vi "comunicacion_arduino_ejemplo.vi"() -> ()   [LabVIEW 2014]
panel:
  out "Waveform Chart":dbl(graph)
  in  "Slide":u8(slide) scale=0.0..255.0
  in  "error in (no error)":errorcluster
  in  "baud rate (9600)":u32=9600
  in  "VISA resource name":refnum<visa-resource-name>
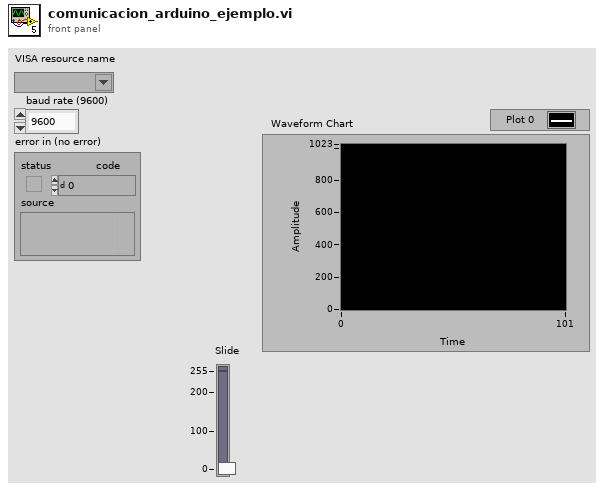
[diagram p1: front panel]
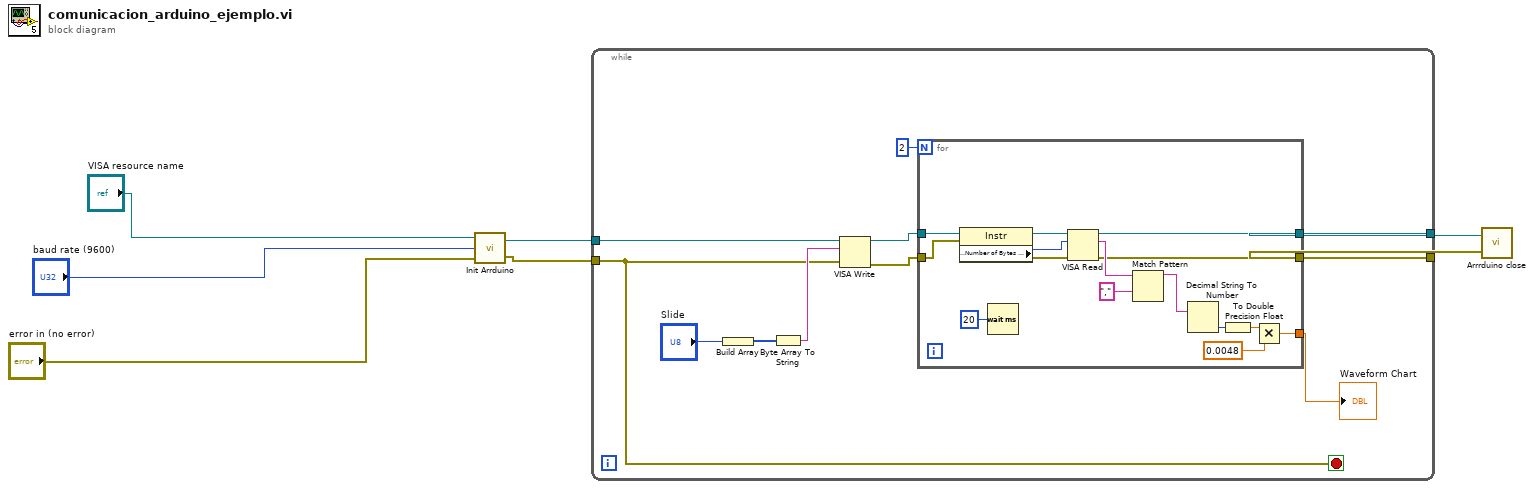
[diagram p0: block diagram]
diagram:
  n1 = call "Init Arrduino.vi"("error in (no error)"="error in (no error)", "baud rate (9600)"="baud rate (9600)", "VISA Refnum in"="VISA resource name") -> ("error out"=w3:errorcluster, "VISA Refnum out"=w4:refnum<visa-resource-name>)
  n2 = while {
    tunnel: w4 -> [w18]
    tunnel: w3 -> [w10]
    tunnel: [w11] -> w2
    tunnel: [w12] -> w1
    stop <- w10 stop-if-true
    n3 = Build Array("Slide") -> (w16:u8[])
    n4 = Byte Array To String(unsigned byte array=w16) -> (string=w15:string)
    n5 = VISA Write(VISA resource name=w18, write buffer=w15, error in (no error)=w10) -> (VISA resource name out=w13:refnum<visa-resource-name>, error out=w14:errorcluster)  [unwired: 1 out]
    n6 = for {
      N: 2 -> [_]
      tunnel: w13 -> [w32]
      tunnel: [w28] -> w12
      tunnel: w14 -> [w33]
      tunnel: [w25] -> w11
      tunnel: [w19] -> w8
      n7 = property class="Instr"(reference=w32, error in=w33) -> (reference out=w31:refnum<visa-resource-name>, error out=w30:errorcluster, "Serial Settings:Number of Bytes at Serial Port"=w29:u32)
      n8 = Wait (ms)(milliseconds to wait=u32 20) -> ()  [unwired: 1 out]
      n9 = VISA Read(VISA resource name=w31, byte count=w29, error in (no error)=w30) -> (VISA resource name out=w28:refnum<visa-resource-name>, read buffer=w27:string, error out=w25:errorcluster)  [unwired: 1 out]
      n10 = Match Pattern(string=w27, regular expression=",") -> (before substring=w24:string)  [unwired: 1 in, 3 out]
      n11 = Decimal String To Number(string=w24) -> (number=w21:i32)  [unwired: 2 in, 1 out]
      n12 = To Double Precision Float(number=w21) -> (double precision float=w22:dbl)
      n13 = Multiply(x=w22, y=0.0048) -> (x*y=w19:dbl)
    }
    "Waveform Chart" <- w8
  }
  n14 = call "Arrrduino close.vi"("error in (no error)"=w2, "VISA Refnum in"=w1) -> ()  [unwired: 1 in]
